vi "FGV SapID & Name.vi"(8 "error in (no error)":errorcluster, 9 "Enum":enum16{"Read", "Write"}(ring)=enum."Write", 10 "Name":string, 11 "SAP ID":string) -> (0 "error out":errorcluster, 2 "SAP ID 2":string, 3 "Name 2":string)   [LabVIEW 2018, in "Application.lvlib"]
uses:
  Application.lvlib
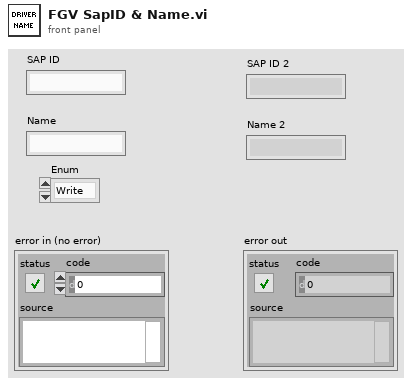
[diagram p1: front panel]
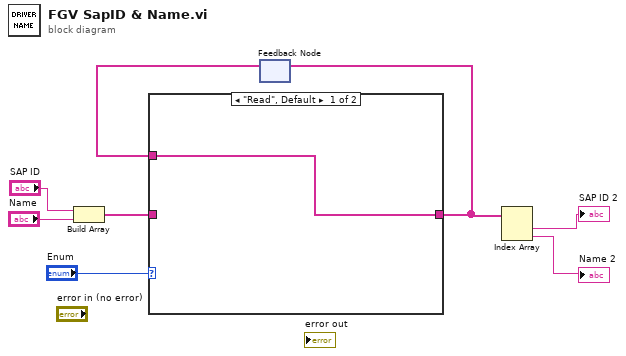
[diagram p0: block diagram]
diagram:
  n1 = Build Array("SAP ID", "Name") -> (w5:string[])
  n2 = feedback #1() -> (w4:string[])  [unwired: 1 in]
  n3 = case shown="\"Read\", Default" "Enum" {
    tunnel: w5 -> [_ w10]
    tunnel: [w9 w10] -> w3
    tunnel: w4 -> [w9 _]
    frame "Read", Default {
    }
    frame "Write" {
    }
  }
  n4 = feedback-in #1(w3) -> ()
  n5 = Index Array(array=w3) -> (element #1=→"SAP ID 2":string, element #2=→"Name 2":string)  [unwired: 2 in]
